vi "IMU.vi"(8 "error in (no error)":errorcluster, 10 "Acc/Gyro  address":u8, 11 "I2C Ref":T1) -> (3 "error out":errorcluster, 5 "IMU Acc":cluster{dbl, dbl, dbl}(graph), 6 "IMU Gyro":cluster{dbl, dbl, dbl}(graph))   [LabVIEW 2019]
uses:
  <vilib>/myRIO/Instrument Drivers/Onboard IO/I2C/typedefs/I2C Reference.ctl
  <vilib>/myRIO/Common/Instrument Driver Framework/Utilities/typedefs/myRIO Generic Hardware Reference.ctl
  <vilib>/myRIO/Common/Instrument Driver Framework/Utilities/typedefs/Hardware Version Enum.ctl
  <vilib>/myRIO/Common/Instrument Driver Framework/Utilities/typedefs/myRIO v1.0 Reference.ctl
  <vilib>/myRIO/Common/Instrument Driver Framework/Utilities/typedefs/Generic FPGA Reference.ctl
  <vilib>/myRIO/Common/Instrument Driver Framework/myRIO v1.0/I2C/typedefs/I2C Channels Enum.ctl
  <vilib>/myRIO/Instrument Drivers/Onboard IO/I2C/typedefs/I2C Configuration.ctl
  <vilib>/myRIO/Instrument Drivers/Onboard IO/I2C/typedefs/I2C Transfer Rate.ctl
  <vilib>/Utility/error.llb/Error Cluster From Error Code.vi
  <vilib>/myRIO/Common/Instrument Driver Framework/myRIO v1.0/I2C/vis/myRIO v1.0 Write I2C.vi
  <vilib>/myRIO/Common/Instrument Driver Framework/myRIO v1.0/I2C/vis/myRIO v1.0 Read I2C.vi
  <vilib>/myRIO/Instrument Drivers/Onboard IO/I2C/I2C.lvlib
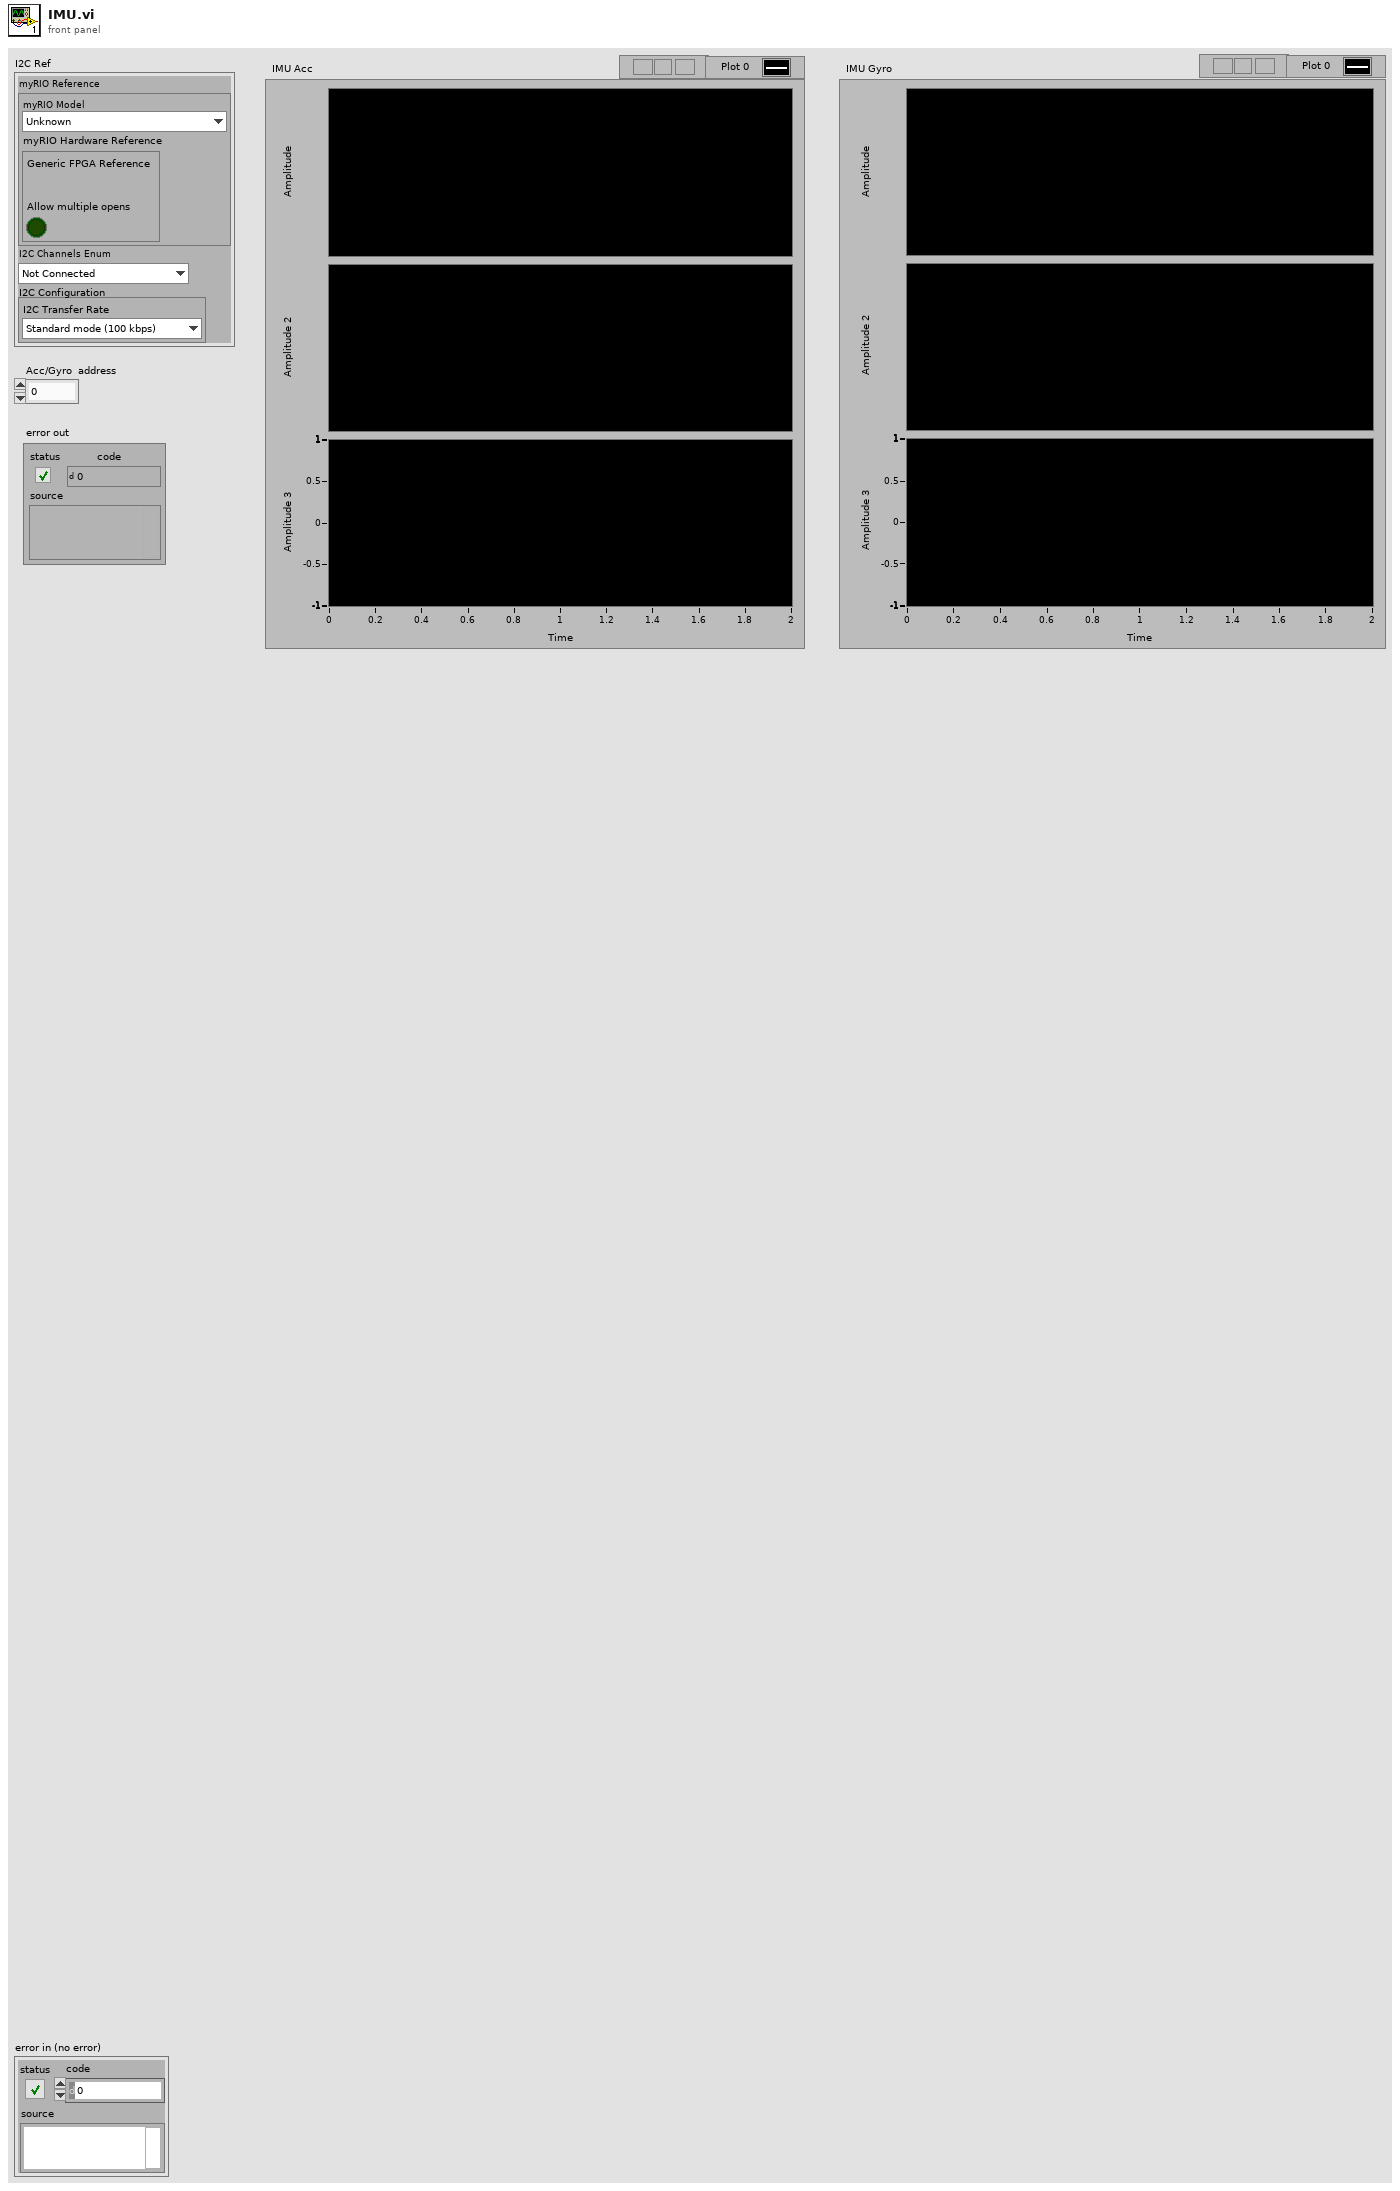
[diagram p1: front panel]
types:
  T1 = typedef "I2C.lvlib/I2C Reference.ctl" = cluster{"myRIO Reference":T2, "I2C Channels Enum":T6, "I2C Configuration":T7}
  T2 = typedef "myRIO Generic Hardware Reference.ctl" = cluster{"myRIO Model":T3, "myRIO Hardware Reference":T4}
  T3 = typedef "Hardware Version Enum.ctl" = enum16{"Unknown", "myRIO-1900", "myRIO-1950", "roboRIO", "NI ELVIS RIO CM", "ELVIS III"}
  T4 = typedef "myRIO v1.0 Reference.ctl" = cluster{"Generic FPGA Reference":T5, "Allow multiple opens":bool}
  T5 = typedef "Generic FPGA Reference.ctl" = refnum<k20>
  T6 = typedef "I2C Channels Enum.ctl" = enum16{"Not Connected", "A/I2C", "B/I2C", "I2C/I2C"}
  T7 = typedef "I2C.lvlib/I2C Configuration.ctl" = cluster{"I2C Transfer Rate":T8}
  T8 = typedef "I2C.lvlib/I2C Transfer Rate.ctl" = enum16{"Standard mode (100 kbps)", "Fast mode (400 kbps)"}
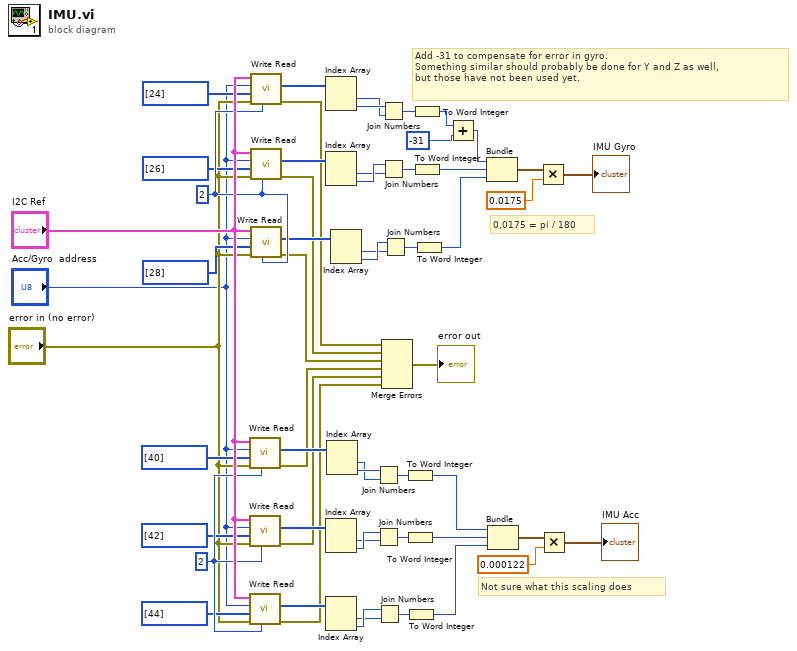
[diagram p0: block diagram]
diagram:
  w41 = u32 2 ("Byte Count")
  w25 = u32 2 ("Byte Count")
  # "Add -31 to compensate for error in gyro.\nSomething similar should probably be done for Y and Z as well,\nbut those have not been used yet."
  # "Not sure what this scaling does"
  # "0,0175 = pi / 180"
  n1 = call <vilib>:"Write Read.vi"("Byte Count"=w25, "error in (no error)"="error in (no error)", "Bytes to Write"=u8[] [40], "Slave Address (7-bit)"="Acc/Gyro  address", "I2C Ref In"="I2C Ref") -> ("error out"=w4:errorcluster, "Bytes Read"=w17:u8[])  [unwired: 3 in, 1 out]
  n2 = call <vilib>:"Write Read.vi"("Byte Count"=w25, "error in (no error)"="error in (no error)", "Bytes to Write"=u8[] [42], "Slave Address (7-bit)"="Acc/Gyro  address", "I2C Ref In"="I2C Ref") -> ("error out"=w3:errorcluster, "Bytes Read"=w15:u8[])  [unwired: 3 in, 1 out]
  n3 = call <vilib>:"Write Read.vi"("Byte Count"=w25, "error in (no error)"="error in (no error)", "Bytes to Write"=u8[] [44], "Slave Address (7-bit)"="Acc/Gyro  address", "I2C Ref In"="I2C Ref") -> ("error out"=w2:errorcluster, "Bytes Read"=w13:u8[])  [unwired: 3 in, 1 out]
  n4 = call <vilib>:"Write Read.vi"("Byte Count"=w41, "error in (no error)"="error in (no error)", "Bytes to Write"=u8[] [24], "Slave Address (7-bit)"="Acc/Gyro  address", "I2C Ref In"="I2C Ref") -> ("error out"=w7:errorcluster, "Bytes Read"=w33:u8[])  [unwired: 3 in, 1 out]
  n5 = call <vilib>:"Write Read.vi"("Byte Count"=w41, "error in (no error)"="error in (no error)", "Bytes to Write"=u8[] [26], "Slave Address (7-bit)"="Acc/Gyro  address", "I2C Ref In"="I2C Ref") -> ("error out"=w6:errorcluster, "Bytes Read"=w31:u8[])  [unwired: 3 in, 1 out]
  n6 = call <vilib>:"Write Read.vi"("Byte Count"=w41, "error in (no error)"="error in (no error)", "Bytes to Write"=u8[] [28], "Slave Address (7-bit)"="Acc/Gyro  address", "I2C Ref In"="I2C Ref") -> ("error out"=w5:errorcluster, "Bytes Read"=w29:u8[])  [unwired: 3 in, 1 out]
  n7 = Index Array "Index Array"(array=w33) -> (element #1=w35:u8, element #2=w36:u8)  [unwired: 2 in]
  n8 = Index Array "Index Array"(array=w31) -> (element #1=w37:u8, element #2=w38:u8)  [unwired: 2 in]
  n9 = Index Array "Index Array"(array=w15) -> (element #1=w21:u8, element #2=w22:u8)  [unwired: 2 in]
  n10 = Index Array "Index Array"(array=w13) -> (element #1=w23:u8, element #2=w24:u8)  [unwired: 2 in]
  n11 = Index Array "Index Array"(array=w17) -> (element #1=w19:u8, element #2=w20:u8)  [unwired: 2 in]
  n12 = Index Array "Index Array"(array=w29) -> (element #1=w39:u8, element #2=w40:u8)  [unwired: 2 in]
  n13 = Join Numbers(hi=w20, lo=w19) -> ((hi.lo)=w10:u16)
  n14 = Join Numbers(hi=w22, lo=w21) -> ((hi.lo)=w11:u16)
  n15 = Join Numbers(hi=w24, lo=w23) -> ((hi.lo)=w12:u16)
  n16 = Join Numbers(hi=w36, lo=w35) -> ((hi.lo)=w26:u16)
  n17 = Join Numbers(hi=w38, lo=w37) -> ((hi.lo)=w27:u16)
  n18 = Join Numbers(hi=w40, lo=w39) -> ((hi.lo)=w28:u16)
  n19 = Merge Errors(w7, w6, w5, w4, w3, w2) -> (→"error out":errorcluster)
  n20 = To Word Integer(number=w10) -> (16bit integer=w51:i16)
  n21 = To Word Integer(number=w11) -> (16bit integer=w50:i16)
  n22 = To Word Integer(number=w12) -> (16bit integer=w49:i16)
  n23 = To Word Integer(number=w26) -> (16bit integer=w53:i16)
  n24 = To Word Integer(number=w27) -> (16bit integer=w47:i16)
  n25 = To Word Integer(number=w28) -> (16bit integer=w48:i16)
  n26 = Add(x=w53, y=-31) -> (x+y=w54:i32)
  n27 = Bundle "Bundle"(w54, w47, w48) -> (w44:cluster{i32, i16, i16})  [unwired: 1 in]
  n28 = Bundle "Bundle"(w51, w50, w49) -> (w43:cluster{i16, i16, i16})  [unwired: 1 in]
  n29 = Multiply(x=w44, y=0.0175) -> (x*y=→"IMU Gyro":cluster{dbl, dbl, dbl})
  n30 = Multiply(x=w43, y=0.000122) -> (x*y=→"IMU Acc":cluster{dbl, dbl, dbl})
